vi "Read demandRADec.vi"(8 "error in (no error)":errorcluster, 11 "PointingPositions in":refnum<class "PointingPositions.lvclass">) -> (0 "error out":errorcluster, 2 "RADecParameters.lvclass":refnum<class "RADecParameters.lvclass">, 3 "PointingPositions out":refnum<class "PointingPositions.lvclass">)   [LabVIEW 2022 SP3, in "TCSDataDefinitions.lvlib" / "TCSPublicStatus.lvlib" / "PointingPositions.lvlib" / "PointingPositions.lvclass"]
uses:
  PointingPositions.lvclass
  TCSCommand/TargetConfiguration/Target/FixedTarget/RADecParameters/RADecParameters.lvclass
  PointingPositions.lvclass/PointingPositions.ctl
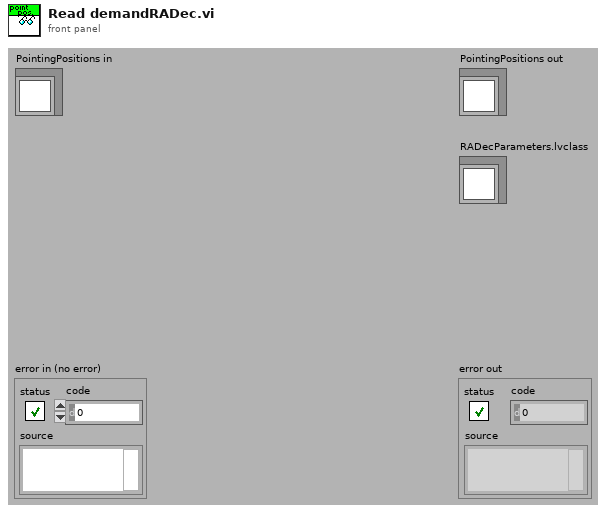
[diagram p1: front panel]
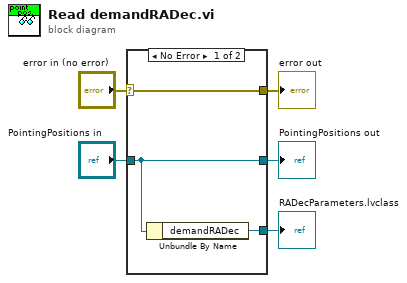
[diagram p0: block diagram]
diagram:
  n1 = case shown="No Error" "error in (no error)" {
    selector: "error in (no error)" -> [w8 w9]
    tunnel: [w8 w9] -> w4
    tunnel: [w7 w10] -> w2
    tunnel: "PointingPositions in" -> [w7 w10]
    tunnel: [w6 _] -> w1
    frame No Error {
      n2 = Unbundle By Name(w7) -> ("demandRADec"=w6:refnum<class "RADecParameters.lvclass">)
    }
    frame Error {
    }
  }
  "error out" <- w4
  "PointingPositions out" <- w2
  "RADecParameters.lvclass" <- w1
